vi "Timeout Notifier Core.vi"(8 "Time To Wait":i32=1000, 9 "Timeout Notifier":refnum<notifier>, 10 "Timeout Action":T1, 11 "Message Cycle Notifier":refnum<notifier>) -> ()   [LabVIEW 2020, in "MessageCycle.lvclass"]
doc: "超时通知核心"
uses:
  MessageCycle.lvclass
  Message Cycle Notifications.ctl
  Timeout Notifications.ctl
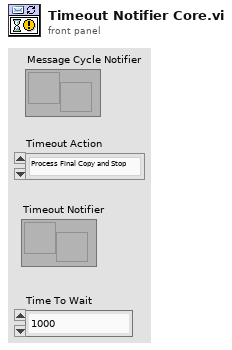
[diagram p1: front panel]
types:
  T1 = typedef "MessageCycle.lvclass/Message Cycle Notifications.ctl" = enum16{"Process Final Copy and Stop", "Stop Immediately", "Substitute Last Message and Stop"}
  T2 = typedef "MessageCycle.lvclass/Timeout Notifications.ctl" = enum16{"Cancel Timeout", "Force Timeout"}
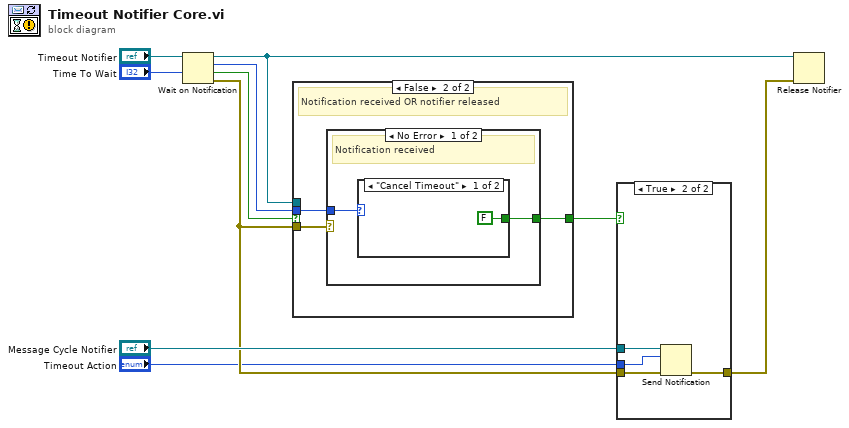
[diagram p0: block diagram]
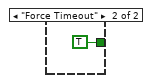
[diagram p3: hidden frame]
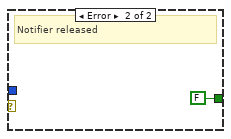
[diagram p4: hidden frame]
diagram:
  n1 = Wait on Notification(notifier="Timeout Notifier", timeout in ms (-1)="Time To Wait") -> (notifier out=w2:refnum<notifier>, notification=w3:T2, timed out?=w5:bool, error out=w6:errorcluster)  [unwired: 2 in]
  n2 = case shown="False" w5 {
    selector: w5 -> [w11 _]
    tunnel: [w11 w13] -> w4
    tunnel: w3 -> [_ w12]
    tunnel: w6 -> [_ w14]
    tunnel: w2 -> [_ _]
    frame True {
      # "Timed out -- Send notification"
    }
    frame False {
      # "Notification received OR notifier released"
      n3 = case shown="No Error" w14 {
        tunnel: [w15 FALSE] -> w13
        tunnel: w12 -> [w16 _]
        frame No Error {
          # "Notification received"
          n4 = case shown="\"Cancel Timeout\"" w16 {
            tunnel: [FALSE TRUE] -> w15
            frame "Cancel Timeout" {
            }
            frame "Force Timeout" {
            }
          }
        }
        frame Error {
          # "Notifier released"
        }
      }
    }
  }
  n5 = case shown="True" w4 {
    tunnel: "Message Cycle Notifier" -> [_ w22]
    tunnel: "Timeout Action" -> [_ w21]
    tunnel: w6 -> [w20 w24]
    tunnel: [w20 w23] -> w8
    frame False {
    }
    frame True {
      n6 = Send Notification(notification=w21, notifier=w22, error in (no error)=w24) -> (error out=w23:errorcluster)  [unwired: 1 out]
    }
  }
  n7 = Release Notifier(notifier=w2, error in (no error)=w8) -> ()  [unwired: 1 in, 3 out]
